vi "SetRF.vi"(0 "reference in":refnum<class "mmWave instrument.lvclass">, 5 "Port":string(combo), 7 "Frequency":dbl format="%#_6pHz", 9 "Gain":dbl format="%#_6fdb", 11 "error in (no error)":errorcluster) -> (4 "reference out":refnum<class "mmWave instrument.lvclass">, 15 "error out":errorcluster)   [LabVIEW 2019, in "mmWave instrument.lvclass"]
doc: "Set RF configuration for port:\nGain and frequency"
uses:
  mmWave instrument.lvclass
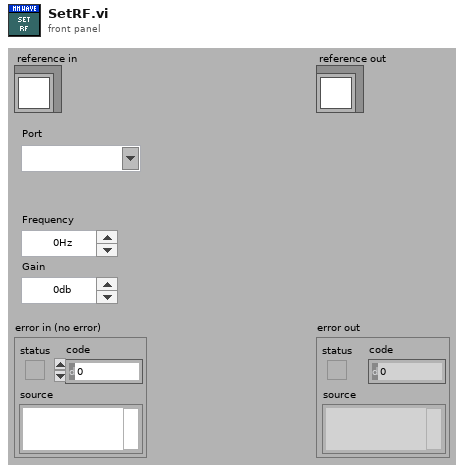
[diagram p1: front panel]
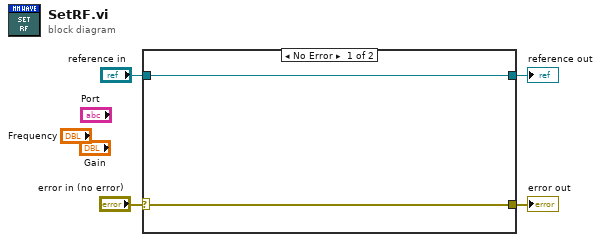
[diagram p0: block diagram]
diagram:
  n1 = case shown="No Error" "error in (no error)" {
    selector: "error in (no error)" -> [w5 w8]
    tunnel: [w5 w8] -> w3
    tunnel: [w6 w7] -> w1
    tunnel: "reference in" -> [w6 w7]
    frame No Error {
    }
    frame Error {
    }
  }
  "error out" <- w3
  "reference out" <- w1
